vi "CamGetImage.vi"(8 "error in (no error)":errorcluster, 9 "buffer for frame":u16[](array[numeric]), 11 "hCam":i16) -> (0 "error out":errorcluster, 2 "output array":u16[][](array[numeric]), 3 "hCam out":i16)   [LabVIEW 2021]
uses:
  LabVIEW.exe
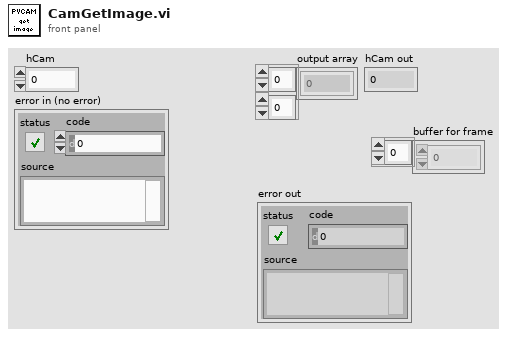
[diagram p1: front panel]
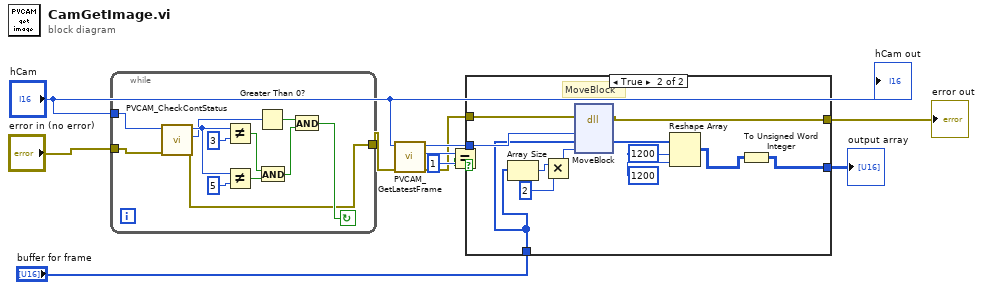
[diagram p0: block diagram]
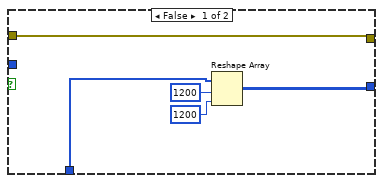
[diagram p2: hidden frame]
diagram:
  n1 = while {
    tunnel: [w16] -> w4
    tunnel: "hCam" -> [w15]
    tunnel: "error in (no error)" -> [w14]
    stop <- w17 continue-if-true
    n2 = call "PVCAM_CheckContStatus.vi"("error in (no error)"=w14, "hCam"=w15) -> ("error out"=w16:errorcluster, "return type"=w13:i16, "status"=w22:i16)  [unwired: 5 in, 2 out]
    n3 = Not Equal?(x=w22, y=i16 3) -> (x != y?=w20:bool)
    n4 = Not Equal?(x=w22, y=i16 5) -> (x != y?=w19:bool)
    n5 = Greater Than 0?(x=w13) -> (x > 0?=w12:bool)
    n6 = And(x=w20, y=w19) -> (x .and. y?=w18:bool)
    n7 = And(x=w12, y=w18) -> (x .and. y?=w17:bool)
  }
  n8 = call "PVCAM_GetLatestFrame.vi"("error in (no error)"=w4, "hCam"="hCam") -> ("error out"=w3:errorcluster, "return"=w9:i16, "frame ptr"=w10:u64)  [unwired: 6 in]
  n9 = Equal?(x=w9, y=i16 1) -> (x = y?=w7:bool)
  n10 = case shown="True" w7 {
    tunnel: w10 -> [_ w38]
    tunnel: [w28 w33] -> w6
    tunnel: w3 -> [w25 w36]
    tunnel: [w25 w35] -> w5
    tunnel: "buffer for frame" -> [w24 w32]
    frame False {
      n11 = Reshape Array(w24, 1200 ("dimension size"), 1200 ("dimension size")) -> (w28:u16[][])
    }
    frame True {
      # "MoveBlock"
      n12 = Array Size(array=w32) -> (size(s)=w31:i32)
      n13 = Multiply(x=w31, y=2) -> (x*y=w30:i32)
      n14 = dll-call lib="LabVIEW.exe" fn="MoveBlock"(error in=w36, "source"=w38, "dest"=w32, "size"=w30) -> (error out=w35:errorcluster, "dest"=w37:u16[])  [unwired: 5 in, 1 out]
      n15 = Reshape Array(w37, 1200 ("dimension size"), 1200 ("dimension size")) -> (w34:u16[][])
      n16 = To Unsigned Word Integer(number=w34) -> (unsigned 16bit integer=w33:u16[][])
    }
  }
  "output array" <- w6
  "error out" <- w5
  "hCam out" <- "hCam"
